vi "Init.vi"(8 "error in (no error)":errorcluster, 11 "TCP Writer in":refnum<class "TCP Writer.lvclass">) -> (0 "error out":errorcluster, 3 "TCP Writer out":refnum<class "TCP Writer.lvclass">)   [LabVIEW 2026, in "TALOS.lvlib" / "TCP Writer.lvlib" / "TCP Writer.lvclass"]
uses:
  TCP Writer.lvclass
  C:/LabVIEW Code/TALOS/talos/Ancestor/Ancestor/Ancestor.lvclass
  C:/LabVIEW Code/TALOS/talos/Father of all uServices/Father of all uServices/Father of all uServices.lvclass
  Ancestor/Ancestor/Ancestor.lvclass/Ancestor.ctl
  Father of all uServices/Father of all uServices/Father of all uServices.lvclass/Father of all uServices.ctl
  TCP Writer.lvclass/TCP Writer.ctl
  Support VIs/Substitute Error.vi
  Support VIs/Generate Error.vi
  FGV/Error Memory/Get Error Description.vi
  Support VIs/Get PC name.vi
  Support VIs/Get Class Name.vi
  <vilib>/Utility/error.llb/Clear Errors.vi
  FGV/Error Memory/Error Memory Core.vi
  <vilib>/AdvancedString/Delimited String to 1D String Array.vi
  <vilib>/AdvancedString/Delimited String to 1D String Array (string).vi
  Support VIs/Circus Root Path.vi
  FGV/Error Memory/Error Crt Lvl checker.vi
  FGV/Error Memory/Error Memory Core.vi/40c8088d-b597-4017-91af-faa98e00292e.vi
  FGV/Error Memory/Error Memory Core.vi/d4a3ab98-063c-4e44-b43d-fbdcfe6c2be2.vi
  Support VIs/Global Memory.vi
  <vilib>/Utility/LVClass/Get LV Class Name.vi
  Support VIs/Is in Packed Library.vi
  Support VIs/TALOS Root path.vi
  Support VIs/Read CSV worksheet.vi
  Support VIs/Global Constants.vi
  <vilib>/Utility/error.llb/General Error Handler.vi
  Support VIs/Error Log.vi
  Father of all uServices/Father of all uServices/Father of all uServices.lvclass
  Ancestor/Ancestor/Ancestor.lvclass
  <vilib>/Comparison/Equal/Equal Functor/Equal Functor.lvclass
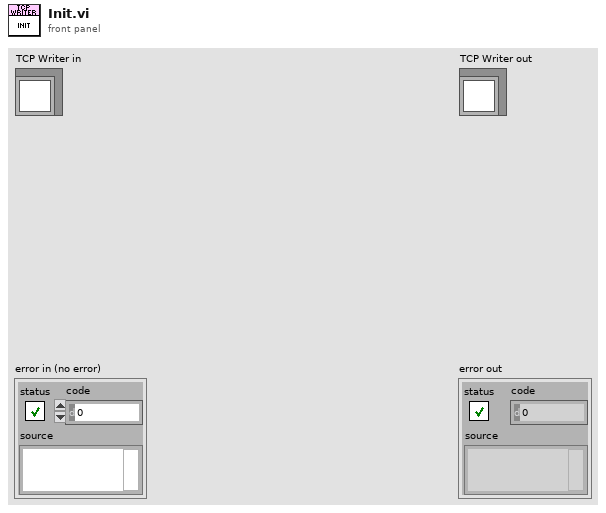
[diagram p1: front panel]
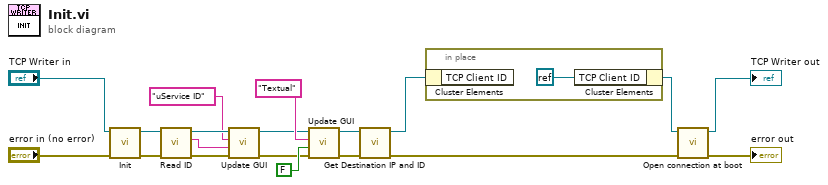
[diagram p0: block diagram]
diagram:
  n1 = call-parent "Init.vi"("error in (no error)"="error in (no error)", "uService Template in"="TCP Writer in") -> ("error out"=w16:errorcluster, "uService Template out"=w17:refnum<class "TCP Writer.lvclass">)  [unwired: 8 in]
  n2 = call "Read ID.vi"("error in (no error)"=w16, "Ancestor in"=w17) -> ("error out"=w15:errorcluster, "ID"=w12:string, "Ancestor out"=w14:refnum<class "TCP Writer.lvclass">)  [unwired: 7 in]
  n3 = call "Update GUI.vi"("error in (no error)"=w15, "Data"=w12, "GUI Item Name"="uService ID", "uService Template in"=w14) -> ("error out"=w7:errorcluster, "uService Template out"=w8:refnum<class "TCP Writer.lvclass">)  [unwired: 6 in]
  n4 = call "Update GUI.vi"("error in (no error)"=w7, "Data"=FALSE ("Textual"), "GUI Item Name"="Textual", "uService Template in"=w8) -> ("error out"=w6:errorcluster, "uService Template out"=w5:refnum<class "TCP Writer.lvclass">)  [unwired: 6 in]
  n5 = call-dynamic "Get Destination IP and ID.vi"("error in (no error)"=w6, "TCP Writer in"=w5) -> ("error out"=w2:errorcluster, "TCP Writer out"=w11:refnum<class "TCP Writer.lvclass">)  [unwired: 8 in]
  n6 = in-place {
    n7 = in-place-cluster #1(w11) -> ()  [unwired: 1 out]
    n8 = in-place-cluster #1("TCP Client ID"=refnum<k0> refnum) -> (w4:refnum<class "TCP Writer.lvclass">)
  }
  n9 = call-dynamic "Open connection at boot.vi"("error in (no error)"=w2, "TCP Writer in"=w4) -> ("error out"=→"error out":errorcluster, "TCP Writer out"=→"TCP Writer out":refnum<class "TCP Writer.lvclass">)  [unwired: 8 in]
